vi "Calculate Driving Direction of Tank1_0713.vi"(8 "error in (no error)":errorcluster, 10 "obstacle angles (rad)":dbl[](array[numeric]), 11 "obstacle distances (m)":dbl[](array[numeric])) -> (0 "error out":errorcluster, 3 "steering frame velocity":dbl[](array[numeric]))   [LabVIEW 2012]
doc: "Calculates the velocity vector of the robot required to avoid obstacles, based on the scanned data."
uses:
  <vilib>/robotics/Obstacle Avoidance/Simple Vector Field Histogram/Panic Range.ctl
  <vilib>/Utility/AngleManip/Degrees to Radians (Scalar DBL).vi
  <vilib>/robotics/Obstacle Avoidance/Simple Vector Field Histogram/NI_Robotics_Simple Vector Field Histogram.lvlib
  <vilib>/Utility/AngleManip/NI_AngleManipulation.lvlib
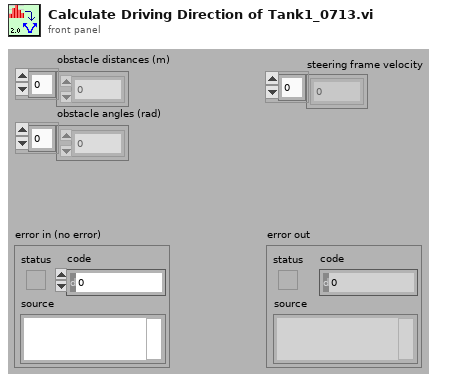
[diagram p1: front panel]
types:
  T1 = typedef "NI_Robotics_Simple Vector Field Histogram.lvlib/Panic Range.ctl" = cluster{"panic threshold distance (0)":dbl, "panic threshold angle (0)":dbl}
  T2 = typedef "NI_Robotics_Simple Vector Field Histogram.lvlib/Obstacle Description.ctl" = cluster{"angle to obstacle":dbl, "distance to obstacle":dbl}
  T3 = typedef "NI_Robotics_Simple Vector Field Histogram.lvlib/Gap Description.ctl" = cluster{"angle to gap":dbl, "size of gap":dbl}
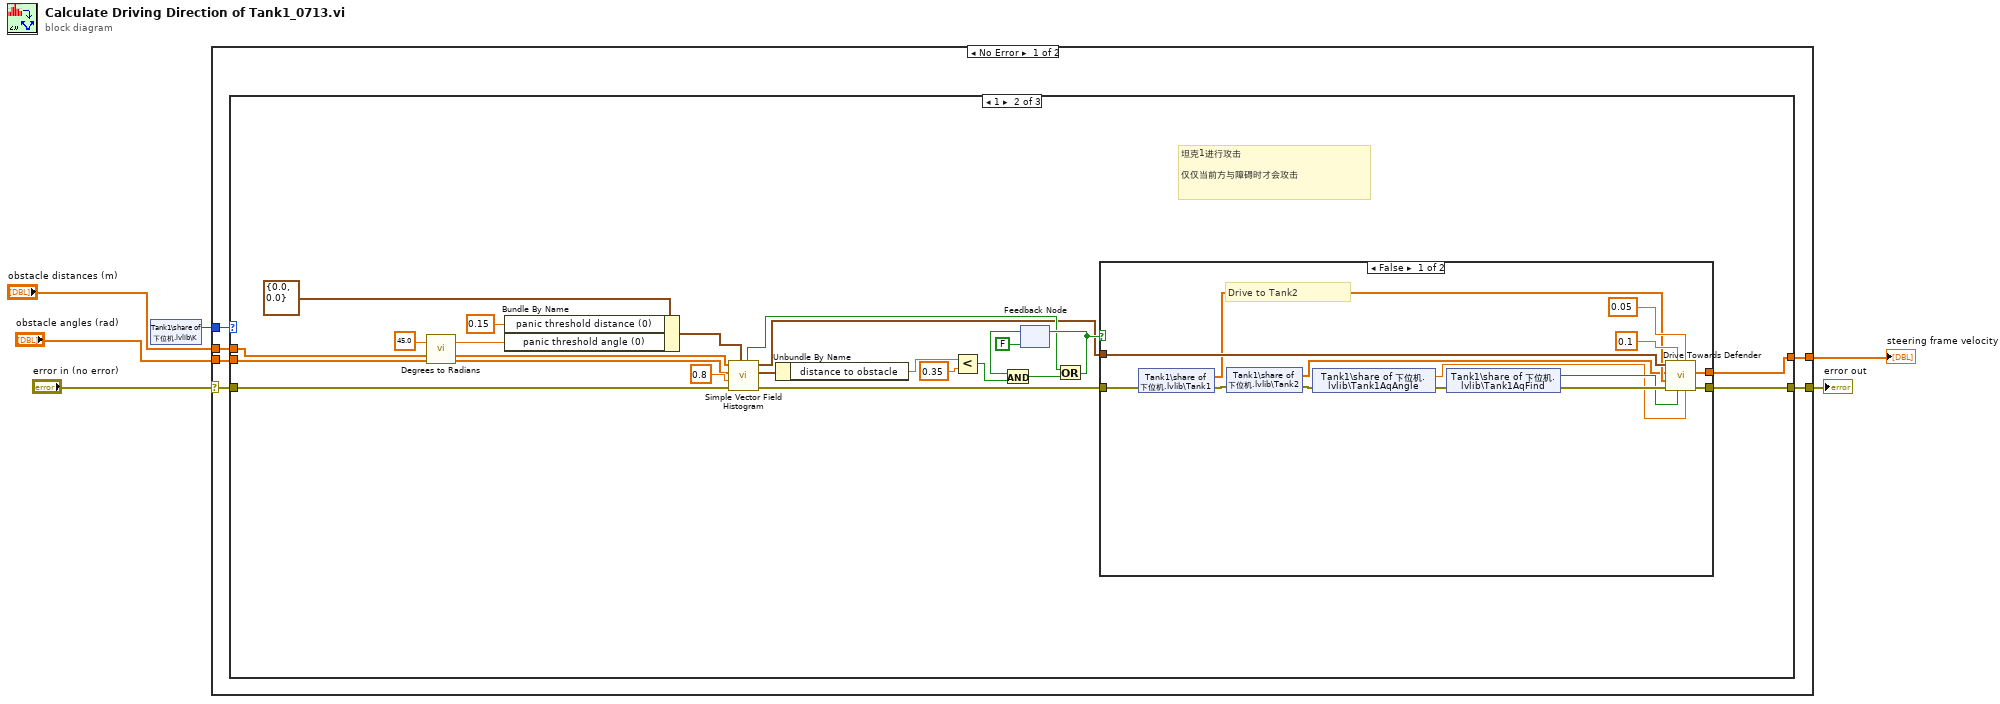
[diagram p0: block diagram]
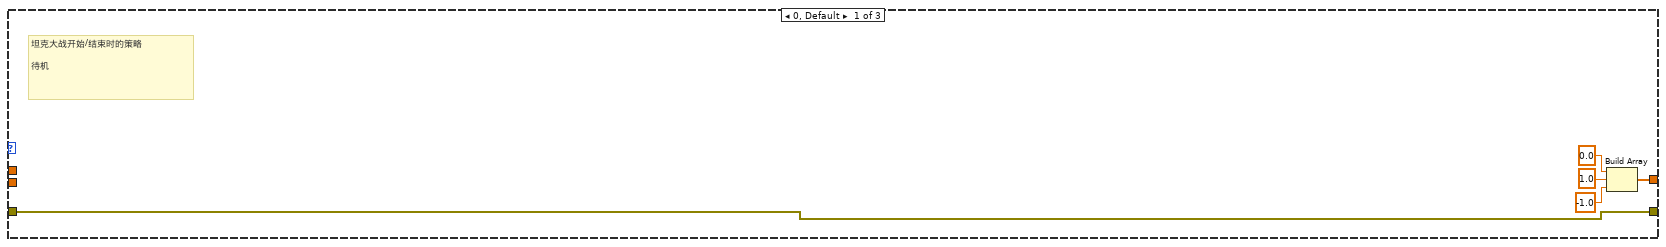
[diagram p2: hidden frame]
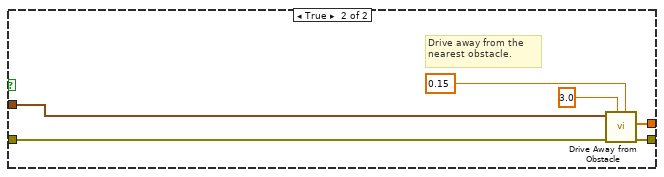
[diagram p3: hidden frame]
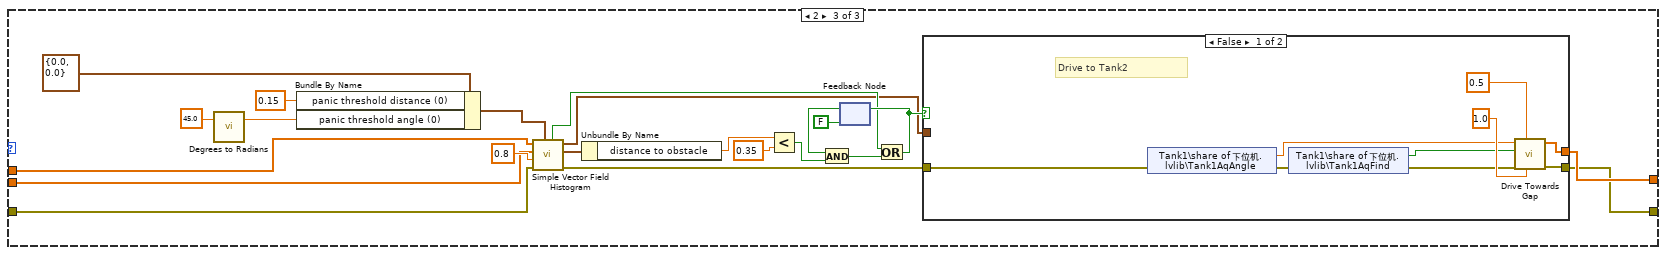
[diagram p4: hidden frame]
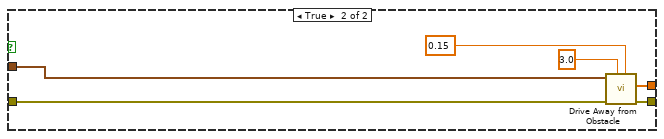
[diagram p5: hidden frame]
diagram:
  n1 = shared-variable "Tank1\\share of 下位机.lvlib\\K"() -> (w1:i16)  [unwired: 1 in, 1 out]
  n2 = case shown="No Error" "error in (no error)" {
    selector: "error in (no error)" -> [w11 w97]
    tunnel: [w12 w97] -> w6
    tunnel: "obstacle distances (m)" -> [w10 _]
    tunnel: "obstacle angles (rad)" -> [w9 _]
    tunnel: [w8 _] -> w2
    tunnel: w1 -> [w7 _]
    frame No Error {
      n3 = case shown="1" w7 {
        tunnel: [w13 w23 w60] -> w12
        tunnel: w11 -> [w13 w22 w64]
        tunnel: w10 -> [_ w21 w62]
        tunnel: w9 -> [_ w18 w63]
        tunnel: [w14 w20 w61] -> w8
        frame 0, Default {
          # "坦克大战开始/结束时的策略\n\n待机"
          n4 = Build Array(0.0 ("panic threshold angle (rad)"), 1.0 ("distance threshold (m)"), -1.0 ("distance threshold (m)")) -> (w14:dbl[])
        }
        frame 1 {
          # "坦克1进行攻击\n\n仅仅当前方与障碍时才会攻击"
          n5 = call-poly <vilib>:"Degrees to Radians.vi"("angle (deg)"=45.0 ("panic threshold angle (rad)")) -> ("angle (rad)"=w39:dbl)  [unwired: 2 in]
          n6 = Bundle By Name(cluster=T1 {"panic threshold distance (0)"=0.0, "panic threshold angle (0)"=0.0} ("panic range"), "panic threshold distance (0)"=0.15 ("panic threshold distance (m)"), "panic threshold angle (0)"=w39) -> (w27:T1)
          n7 = call <vilib>:"Simple Vector Field Histogram.vi"("panic range"=w27, "error in (no error)"=w22, "distance threshold"=0.8 ("distance threshold (m)"), "direction angles"=w18, "distances"=w21) -> ("error out"=w24:errorcluster, "nearest obstacle"=w29:T2, "largest gap"=w19:T3, "obstacle within panic range"=w34:bool)  [unwired: 2 in, 1 out]
          n8 = Unbundle By Name(w29) -> ("distance to obstacle"=w30:dbl)
          n9 = Less?(x=w30, y=0.35) -> (x < y?=w32:bool)
          n10 = feedback #1(FALSE ("obstacle within panic range")) -> (w33:bool)
          n11 = And(x=w33, y=w32) -> (x .and. y?=w35:bool)
          n12 = Or(x=w34, y=w35) -> (x .or. y?=w37:bool)
          n13 = feedback-in #1(w37) -> ()
          n14 = case shown="False" w37 {
            tunnel: w19 -> [w53 w57]
            tunnel: w24 -> [w47 w59]
            tunnel: [w52 w58] -> w23
            tunnel: [w51 w56] -> w20
            frame False {
              # "Drive to Tank2"
              n15 = shared-variable "Tank1\\share of 下位机.lvlib\\Tank1"(error in=w47) -> (w46:dbl[], error out=w48:errorcluster)
              n16 = shared-variable "Tank1\\share of 下位机.lvlib\\Tank2"(error in=w48) -> (w45:dbl[], error out=w44:errorcluster)
              n17 = shared-variable "Tank1\\share of 下位机.lvlib\\Tank1AqAngle"(error in=w44) -> (w40:dbl, error out=w43:errorcluster)
              n18 = shared-variable "Tank1\\share of 下位机.lvlib\\Tank1AqFind"(error in=w43) -> (w41:bool, error out=w42:errorcluster)
              n19 = call "Drive Towards Defender.vi"("defencer angle"=w40, "max forward velocity (m/s)"=0.05, "find"=w41, "max angular velocity (rad/s)"=0.1, "error in (no error)"=w42, "attacker"=w46, "defender"=w45, "gap"=w53) -> ("error out"=w52:errorcluster, "steering frame velocity"=w51:dbl[])  [unwired: 2 in]
            }
            frame True {
              # "Drive away from the nearest obstacle."
              n20 = call "Drive Away from Obstacle.vi"("max reverse velocity (m/s)"=0.15, "max angular velocity (rad/s)"=3.0, "error in (no error)"=w59, "gap"=w57) -> ("error out"=w58:errorcluster, "steering frame velocity"=w56:dbl[])  [unwired: 6 in]
            }
          }
        }
        frame 2 {
          n21 = call-poly <vilib>:"Degrees to Radians.vi"("angle (deg)"=45.0 ("panic threshold angle (rad)")) -> ("angle (rad)"=w81:dbl)  [unwired: 2 in]
          n22 = Bundle By Name(cluster=T1 {"panic threshold distance (0)"=0.0, "panic threshold angle (0)"=0.0} ("panic range"), "panic threshold distance (0)"=0.15 ("panic threshold distance (m)"), "panic threshold angle (0)"=w81) -> (w69:T1)
          n23 = call <vilib>:"Simple Vector Field Histogram.vi"("panic range"=w69, "error in (no error)"=w64, "distance threshold"=0.8 ("distance threshold (m)"), "direction angles"=w63, "distances"=w62) -> ("error out"=w66:errorcluster, "nearest obstacle"=w71:T2, "largest gap"=w65:T3, "obstacle within panic range"=w76:bool)  [unwired: 2 in, 1 out]
          n24 = Unbundle By Name(w71) -> ("distance to obstacle"=w72:dbl)
          n25 = Less?(x=w72, y=0.35) -> (x < y?=w74:bool)
          n26 = feedback #2(FALSE ("obstacle within panic range")) -> (w75:bool)
          n27 = And(x=w75, y=w74) -> (x .and. y?=w77:bool)
          n28 = Or(x=w76, y=w77) -> (x .or. y?=w79:bool)
          n29 = feedback-in #2(w79) -> ()
          n30 = case shown="False" w79 {
            tunnel: w65 -> [_ w94]
            tunnel: w66 -> [w82 w96]
            tunnel: [w89 w95] -> w60
            tunnel: [w83 w93] -> w61
            frame False {
              # "Drive to Tank2"
              n31 = shared-variable "Tank1\\share of 下位机.lvlib\\Tank1AqAngle"(error in=w82) -> (w84:dbl, error out=w90:errorcluster)
              n32 = shared-variable "Tank1\\share of 下位机.lvlib\\Tank1AqFind"(error in=w90) -> (w86:bool, error out=w85:errorcluster)
              n33 = call "Drive Towards Gap.vi"("max angular velocity (rad/s)"=1.0, "max reverse velocity (m/s)"=0.5 ("max forward velocity (m/s)"), "error in (no error)"=w85, "findA"=w86, "angle"=w84) -> ("error out"=w89:errorcluster, "steering frame velocity"=w83:dbl[])  [unwired: 5 in]
            }
            frame True {
              n34 = call "Drive Away from Obstacle.vi"("max reverse velocity (m/s)"=0.15, "max angular velocity (rad/s)"=3.0, "error in (no error)"=w96, "gap"=w94) -> ("error out"=w95:errorcluster, "steering frame velocity"=w93:dbl[])  [unwired: 6 in]
            }
          }
        }
      }
    }
    frame Error {
    }
  }
  "error out" <- w6
  "steering frame velocity" <- w2
